vi "View DB alarms.vi"(7 "ActivateALRView":bool, 11 "Alarms in":T1) -> (2 "Reread out":bool)   [LabVIEW 2019, in "Alarms.lvlib"]
uses:
  Alarms.lvlib
  Ctl/ALR type.ctl
  Ctl/ALR code.ctl
  Ctl/Alarms.ctl
  Ctl/ALR_defs.ctl
  Ctl/ALRs_State.ctl
  Ctl/ALR_ON_OFF.ctl
  Ctl/ALR_Parameters.ctl
  Database/Progress.vi
  Database/PostgreSQL.lvlib
  Logik/Logik.lvlib
panel:
  out "AI progress":i32(slide) scale=0.0..100.0
  in  "Reread":bool
  in  "n_elem":i32(c297)
  out "Names table":string[](array[string])=["", "Перелив в емкости охлажденной воды", "Уровень в емкости охлажденной воды низкий", "Уровень в емкости охлажденной воды аварийно низкий", "Датчик уровня в емкости охлажденной воды неисправен", "Давление после насосов градирни аварийно высокое", "Давление после насосов градирни высокое", "Давление после насосов градирни низкое", "Давление после насосов градирни аварийно низкое", "Датчик давления после насосов градирни неисправен", "Давление перед градирней аварийно высокое", "Давление перед градирней высокое", "Давление перед градирней низкое", "Давление перед градирней аварийно низкое", "Датчик давления перед градирней неисправен", "Перелив в емкости дистиллята", "Уровень в емкости дистиллята низкий", "Уровень в емкости дистиллята аварийно низкий", "Датчик уровеня в емкости дистиллята неисправен", "Давление после насосов дистиллята низкое", "Давление после насосов дистиллята аварийно низкое", "Датчик давления после насосов дистиллята неисправен", "Давление дистиллята перед реактором низкое", "Давление дистиллята перед реактором аварийно низкое", "Датчик давления перед реактором неисправен", "Давление после насоса агломератора низкое", "Давление после насоса агломератора аварийно низкое", "Датчик давления после насоса агломератора неисправен", "Температура после градирни низкая", "Датчик температуры после градирни неисправен", "Датчик температуры перед градирней неисправен", "Датчик температуры дистиллята после насосов неисправен", "Температура дистиллята перед реактором высокая"]
  out "alrtype":T4[](array[typedef])
  out "fcodealr":T5[](array[typedef])
  out "Parameters table":u32[][](array[numeric])=[[0, 0, 0, 0, 0, 0, 0], [1, 11, 5000, 5000, 0, 0, 3], [2, 11, 5000, 5000, 0, 2, 3], [3, 11, 5000, 5000, 0, 3, 3], [4, 11, 1000, 0, 0, 4, 0], [5, 1, 5000, 5000, 0, 1, 3], [6, 1, 5000, 5000, 0, 0, 3], [7, 1, 5000, 5000, 0, 2, 3], [8, 1, 5000, 30000, 0, 3, 3], [9, 1, 1000, 0, 0, 4, 0], [10, 2, 5000, 5000, 0, 1, 3], [11, 2, 5000, 5000, 0, 0, 3], [12, 2, 5000, 5000, 0, 2, 3], [13, 2, 5000, 30000, 0, 3, 3], [14, 2, 1000, 0, 0, 4, 0], [15, 10, 5000, 5000, 0, 0, 3], [16, 10, 5000, 5000, 0, 2, 3], [17, 10, 5000, 5000, 0, 3, 3], [18, 10, 1000, 0, 0, 4, 0], [19, 3, 5000, 5000, 0, 2, 3], [20, 3, 5000, 5000, 0, 3, 3], [21, 3, 1000, 0, 0, 4, 0], [22, 4, 5000, 5000, 0, 2, 3], [23, 4, 5000, 5000, 0, 3, 3], [24, 4, 1000, 0, 0, 4, 0], [25, 5, 5000, 5000, 0, 2, 3], [26, 5, 5000, 5000, 0, 3, 3], [27, 5, 1000, 0, 0, 4, 0], [28, 6, 5000, 5000, 0, 2, 3], [29, 6, 1000, 0, 0, 4, 0], [30, 7, 1000, 0, 0, 4, 0], [31, 8, 1000, 0, 0, 4, 0], [32, 9, 5000, 5000, 0, 0, 3]]
  out "parameters":string[](array[string])=["", "H1.EP.CL2.BL1", "H1.EP.CL2.BL1", "H1.EP.CL2.BL1", "H1.EP.CL2.BL1", "H1.EP.BP1", "H1.EP.BP1", "H1.EP.BP1", "H1.EP.BP1", "H1.EP.BP1", "H1.EP.BP2", "H1.EP.BP2", "H1.EP.BP2", "H1.EP.BP2", "H1.EP.BP2", "H1.EP.CL1.BL1", "H1.EP.CL1.BL1", "H1.EP.CL1.BL1", "H1.EP.CL1.BL1", "H1.EP.BP3", "H1.EP.BP3", "H1.EP.BP3", "H1.EP.BP4", "H1.EP.BP4", "H1.EP.BP4", "H1.EP.BP5", "H1.EP.BP5", "H1.EP.BP5", "H1.EP.BT1", "H1.EP.BT1", "H1.EP.BT2", "H1.EP.BT3", "H1.EP.BT4"]
  out "n alr":i32
  # "fnum"
  # "alr_ton"
  # "alr_toff"
  # "n_repeat"
  # "fcodealr"
  # "alr_type"
  # "alr_name"
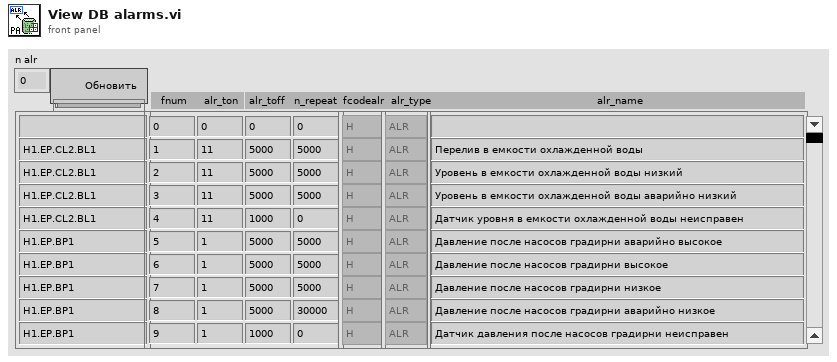
[diagram p1: front panel]
types:
  T1 = typedef "Alarms.lvlib/Alarms.ctl" = cluster{"N_param":i32, "ALR_defs":T2, "ALR_State":T3, "ALR_ON_OFF_modified":refnum<data-value>, "ALR_ON_OFF":refnum<data-value>, "ALRP_modified":refnum<data-value>, "ALRP":refnum<data-value>, "ALRNames":refnum<data-value>}
  T2 = typedef "Alarms.lvlib/ALR_defs.ctl" = cluster{"N_repeat":u32[], "Delay_R":cluster{"not in":bool, "T old":u32, "out":bool, "Q":bool}[]}
  T3 = typedef "Alarms.lvlib/ALRs_State.ctl" = cluster{"ALR not block":bool[], "ALR":bool[], "ALR blocked":bool[], "ALR ON":bool[], "code":i32[], "level":i32[][], "t ms":u32[], "ack state":enum32{"not", "tripped", "reset", "ack"}[], "color":u32[]}
  T4 = typedef "Alarms.lvlib/ALR type.ctl" = enum16{"ACD", "ACDR", "ALRN", "ALR"}
  T5 = typedef "Alarms.lvlib/ALR code.ctl" = enum16{"CONN", "H", "HH", "L", "LL", "SERR", "ON", "OFF", "XM19", "XM24", "XM47", "XM51", "XM52", "XM53", "XM54", "XM55", "XM56", "XM61", "XM62", "XM63", "XM64", "XM65", "XM66"}
  T6 = enum32{"Invalid", "Standard", "Closed", "Hidden", "Minimized", "Maximized"}
  T7 = typedef "Alarms.lvlib/ALR_Parameters.ctl" = cluster{"ALR code":T5[], "ALR type":T4[], "ALRParam":u32[][]}
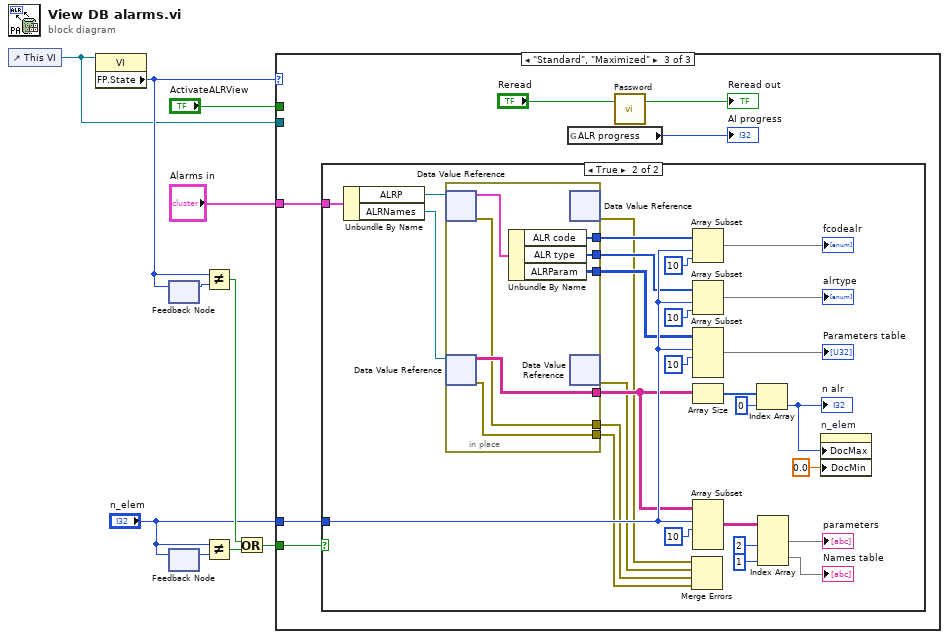
[diagram p0: block diagram]
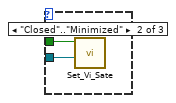
[diagram p3: hidden frame]
diagram:
  n1 = control-ref of="This VI"() -> (w2:refnum<vi>)
  n2 = property class="VI"(reference=w2) -> ("FP.State"=w3:T6)  [unwired: 1 in, 2 out]
  n3 = feedback #1() -> (w9:T6)  [unwired: 1 in]
  n4 = feedback-in #1(w3) -> ()
  n5 = feedback #2() -> (w10:i32)  [unwired: 1 in]
  n6 = feedback-in #2("n_elem") -> ()
  n7 = Not Equal?(x=w3, y=w9) -> (x != y?=w8:bool)
  n8 = Not Equal?(x="n_elem", y=w10) -> (x != y?=w7:bool)
  n9 = Or(x=w8, y=w7) -> (x .or. y?=w6:bool)
  n10 = case shown="\"Standard\", \"Maximized\"" w3 {
    tunnel: "ActivateALRView" -> [_ w11 _]
    tunnel: w2 -> [_ w12 _]
    tunnel: "n_elem" -> [_ _ w17]
    tunnel: w6 -> [_ _ w18]
    tunnel: "Alarms in" -> [_ _ w13]
    frame "Invalid", Default {
    }
    frame "Closed".."Minimized" {
      n11 = call "Set_Vi_Sate.vi"("VI"=w12, "Activate (F)"=w11) -> ()  [unwired: 9 in, 1 out]
    }
    frame "Standard", "Maximized" {
      n12 = case shown="True" w18 {
        tunnel: w17 -> [_ w46]
        tunnel: w13 -> [_ w27]
        frame False {
        }
        frame True {
          n13 = Unbundle By Name(w27) -> ("ALRP"=w26:refnum<data-value>, "ALRNames"=w29:refnum<data-value>)
          n14 = in-place {
            in-place-border: [w53] -> w28
            in-place-border: [w52] -> w22
            in-place-border: [w50] -> w25
            in-place-border: [w49] -> w24
            in-place-border: [w48] -> w23
            in-place-border: [w47] -> w20
            n15 = in-place-dvr #3(w26) -> (w51:T7, w47:errorcluster)
            n16 = in-place-dvr #4(w29) -> (w52:string[][], w53:errorcluster)
            n17 = Unbundle By Name(w51) -> ("ALR code"=w50:T5[], "ALR type"=w49:T4[], "ALRParam"=w48:u32[][])
            n18 = in-place-dvr #3() -> (w19:errorcluster)  [unwired: 1 in, 1 out]
            n19 = in-place-dvr #4() -> (w21:errorcluster)  [unwired: 1 in, 1 out]
          }
          n20 = Merge Errors(w19, w21, w20, w28) -> ()  [unwired: 1 out]
          n21 = Array Subset(array=w25, index=w46, length=10) -> (→"fcodealr":T5[])
          n22 = Array Subset(array=w24, index=w46, length=10) -> (→"alrtype":T4[])
          n23 = Array Subset(array=w23, index (row)=w46, length (row)=10 ("length")) -> (→"Parameters table":u32[][])  [unwired: 2 in]
          n24 = Array Size(array=w22) -> (size(s)=w32:i32[])
          n25 = Array Subset(array=w22, index (row)=w46, length (row)=10 ("length")) -> (w42:string[][])  [unwired: 2 in]
          n26 = Index Array(array=w32, index=0) -> (element=w30:i32)
          "n alr" <- w30
          n27 = Index Array(array=w42, index (col) #1=2 ("index"), index (col) #2=1 ("index (col)")) -> (element #1=→"parameters":string[], element #2=→"Names table":string[])  [unwired: 2 in]
          n28 = property on="n_elem" class="Scroll (strict)"("DocMax"=w30, "DocMin"=0.0 ("Data Entry Limits:Minimum")) -> ()  [unwired: 2 in, 2 out]
        }
      }
      n29 = global read "Progress.vi" "ALR progress"() -> (→"AI progress":i32)
      n30 = call "Password.vi"("ActivatePASSWView"="Reread") -> ("enable"=→"Reread out":bool)  [unwired: 1 in, 1 out]
    }
  }
